vi "normalize_ke_data_start.vi"(7 "Raw y data":dbl[](array[numeric])) -> (8 "Normalized y data":dbl[](array[numeric]))   [LabVIEW 2016]
doc: "This subvi normalizes the K E data by dividing each value in the raw array by the largest individual data point, making the maximum value of the output array 1 at that point, scaling the data over the range [0,1].\n\nPaul K Dixon\nP350\nCSUSB Physics"
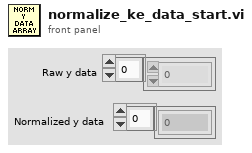
[diagram p1: front panel]
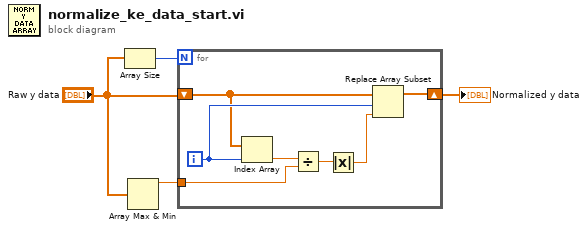
[diagram p0: block diagram]
diagram:
  n1 = Array Size(array="Raw y data") -> (size(s)=w2:i32)
  n2 = Array Max & Min(array="Raw y data") -> (max value=w4:dbl)  [unwired: 3 out]
  n3 = for {
    N: w2 -> [_]
    shift-right: [w10] -> w3
    shift-left: "Raw y data" -> [w8]
    tunnel: w4 -> [w6]
    i -> [w11]
    n4 = Index Array(array=w8, index=w11) -> (element=w7:dbl)
    n5 = Divide(x=w7, y=w6) -> (x/y=w9:dbl)
    n6 = Absolute Value(x=w9) -> (abs(x)=w5:dbl)
    n7 = Replace Array Subset(array=w8, new element=w5, index=w11) -> (w10:dbl[])
  }
  "Normalized y data" <- w3
